vi "Init Server.vi"(7 "Server TLS Config (Disabled)":T1, 8 "error in (no error)":errorcluster, 9 "local-port":u16 caption="incoming-port (0=any)", 10 "Port":u16) -> (0 "error out":errorcluster, 3 "TinyTCP Server":T3)   [LabVIEW 2020, in "TinyTCP.lvlib"]
doc: "Initializes a TCP Server that will listen on the specified server once <b>Open.vi</b> is called. Once Open is called, the server will continually listen for a client to connect and once disconnected will begin listening again. The status of the connection can be checked with <b>Get State.vi</b> Once the connection is no longer needed, call <b>Close.vi</b> to close the server listener and connection if it is connected. To cleanup the client and release all resources call <b>Stop.vi</b>\n\nA Server TLS Config can optionally be specified to enable and enforce TLS handshakes when clients connect. This will cause all data to be encrypted sent via the connection. This requires both the private key and the key's certificate chain. If the private key was encrypted with a password, be sure to specify that as well."
uses:
  TinyTCP.lvlib
  Instance.ctl
  Ref Data.ctl
  State.ctl
  Server TLS Config.ctl
  Cert Chain.ctl
  TLS Config.ctl
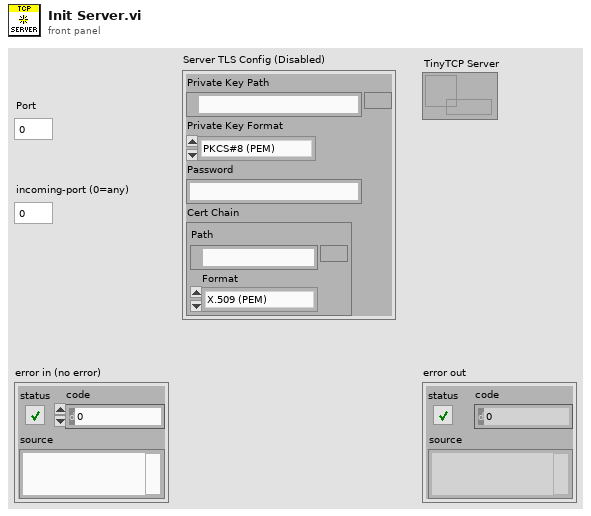
[diagram p1: front panel]
types:
  T1 = typedef "TinyTCP.lvlib/Server TLS Config.ctl" = cluster{"Private Key Path":path, "Private Key Format":enum32{"PKCS#8 (PEM)", "PKCS#8 (DER)"}, "Password":string, "Cert Chain":T2}
  T2 = typedef "TinyTCP.lvlib/Cert Chain.ctl" = cluster{"Path":path, "Format":enum32{"X.509 (PEM)"}}
  T3 = typedef "TinyTCP.lvlib/Instance.ctl" = refnum<data-value>
  T4 = typedef "TinyTCP.lvlib/TLS Config.ctl" = cluster{"TLS Enabled":bool, "Use OS Cert Chains":bool, "Private Key Path":path, "Private Key Format":enum32{"PKCS#8 (PEM)", "PKCS#8 (DER)"}, "Private Key Password":string, "Private Key Cert Chain":T2, "Cert Chains":T2[]}
  T5 = typedef "TinyTCP.lvlib/Ref Data.ctl" = cluster{"TCP":refnum<k5>, "State":T6, "Server":bool, "Host":string, "Port":u16, "Listener":refnum<k5>, "Start":bool, "Disconnect":bool, "TCP Valid":bool, "TLS Enabled":bool, "Immutable TLS":refnum<k36>, "Certificate DN":string, "local-port":u16}
  T6 = typedef "TinyTCP.lvlib/State.ctl" = enum16{"Idle", "Starting", "Connecting", "Connected", "Disconnecting", "Stopped"}
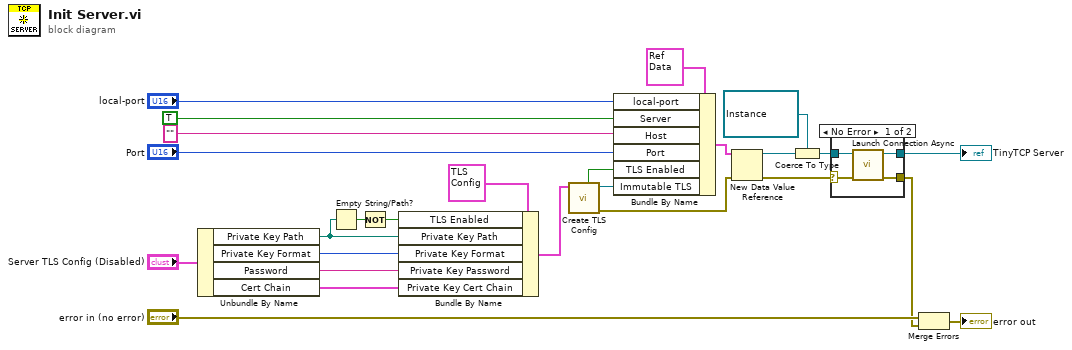
[diagram p0: block diagram]
diagram:
  n1 = Unbundle By Name("Server TLS Config (Disabled)") -> ("Private Key Path"=w8:path, "Private Key Format"=w11:enum32{"PKCS#8 (PEM)", "PKCS#8 (DER)"}, "Password"=w10:string, "Cert Chain"=w9:T2)
  n2 = Empty String/Path?(string/path=w8) -> (empty?=w7:bool)
  n3 = Not(x=w7) -> (.not. x?=w6:bool)
  n4 = Bundle By Name(cluster=T4 {"TLS Enabled"=FALSE, "Use OS Cert Chains"=FALSE, "Private Key Path"=path "", "Private Key Format"=enum."PKCS#8 (PEM)", "Private Key Password"="", "Private Key Cert Chain"={"Path"=path "", "Format"=enum."X.509 (PEM)"}, "Cert Chains"=[]} ("TLS Config"), "TLS Enabled"=w6, "Private Key Path"=w8, "Private Key Format"=w11, "Private Key Password"=w10, "Private Key Cert Chain"=w9) -> (w12:T4)
  n5 = call "Create TLS Config.vi"("TLS Config"=w12) -> ("error out"=w17:errorcluster, "Immutable TLS"=w16:refnum<k36>, "TLS Enabled"=w15:bool)  [unwired: 8 in]
  n6 = Bundle By Name(cluster=T5 {"TCP"=refnum, "State"=enum."Idle", "Server"=FALSE, "Host"="", "Port"=0, "Listener"=refnum, "Start"=FALSE, "Disconnect"=FALSE, "TCP Valid"=FALSE, "TLS Enabled"=FALSE, "Immutable TLS"=refnum, "Certificate DN"="", "local-port"=0} ("Ref Data"), "local-port"="local-port", "Server"=TRUE, "Host"="", "Port"="Port", "TLS Enabled"=w15, "Immutable TLS"=w16) -> (w18:T5)
  n7 = New Data Value Reference(data value=w18, error in=w17) -> (data value reference=w22:refnum<data-value>, error out=w4:errorcluster)
  n8 = Coerce To Type(0:w22, 1:T3 refnum ("TinyTCP Server")) -> (2:w5:T3)
  n9 = case shown="No Error" w4 {
    selector: w4 -> [w28 w31]
    tunnel: w5 -> [w30 w32]
    tunnel: [w29 w32] -> w2
    tunnel: [w27 w31] -> w3
    frame No Error {
      n10 = call "Launch Connection Async.vi"("error in (no error)"=w28, "TCP Comm In"=w30) -> ("error out"=w27:errorcluster, "TCP Comm"=w29:T3)  [unwired: 8 in]
    }
    frame Error {
    }
  }
  "TinyTCP Server" <- w2
  n11 = Merge Errors("error in (no error)", w3) -> (→"error out":errorcluster)
